vi "JTAG Test App.vi"(1 "Stop Button":bool, 8 "Error In":errorcluster, 11 "Device Name":string="Basys2") -> (0 "Error Out":errorcluster, 3 "ID Codes":u32[](array[numeric]) format="%.0x")   [LabVIEW 2011]
uses:
  Private/DMGR/DMGR.lvlib
  Private/DJTG/DJTG.lvlib
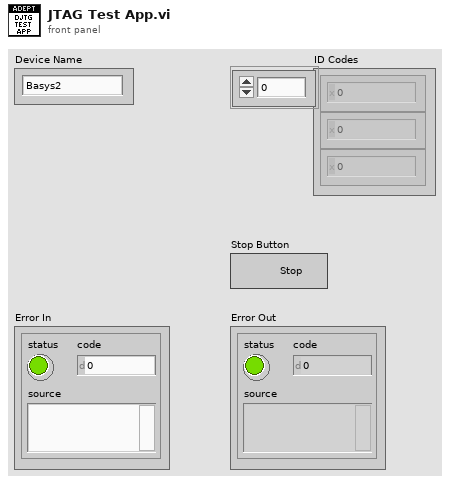
[diagram p1: front panel]
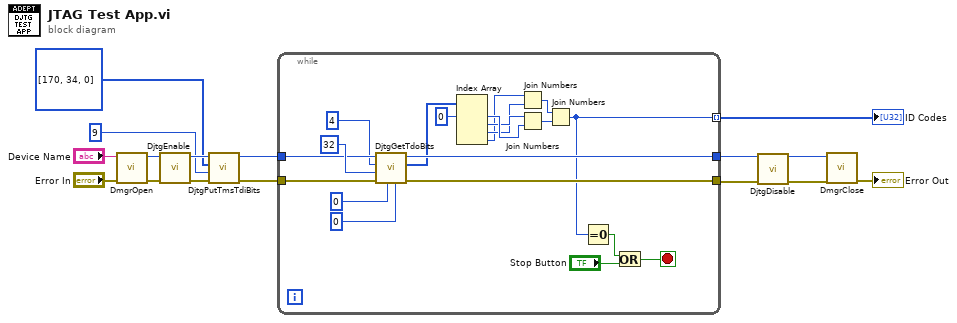
[diagram p0: block diagram]
diagram:
  n1 = call "DmgrOpen.vi"("Error In"="Error In", "Device Name"="Device Name") -> ("Error Out"=w14:errorcluster, "Device Handle"=w13:u32)  [unwired: 8 in]
  n2 = call "DjtgEnable.vi"("Error In"=w14, "Device Number"=w13) -> ("Error Out"=w12:errorcluster, "Device Number"=w11:u32)  [unwired: 8 in]
  n3 = call "DjtgPutTmsTdiBits.vi"("Error In"=w12, "Num Bit Pairs"=u32 9 ("cbitpairs"), "Data To Send"=u8[] [170, 34, 0] ("rgbSnd"), "Device Number"=w11) -> ("Error Out"=w8:errorcluster, "Device Number"=w7:u32)  [unwired: 5 in, 1 out]
  n4 = while {
    tunnel: w8 -> [w36]
    tunnel: w7 -> [w32]
    tunnel: [w31] -> w4
    tunnel: [w30] -> w3
    tunnel: [w20] -> w5 mode=indexing
    stop <- w18 stop-if-true
    n5 = call "DjtgGetTdoBits.vi"("TMS State"=u8 0 ("fTms"), "TDI State"=u8 0 ("fTdi"), "Error In"=w36, "Num Pit Pairs"=u32 32 ("cbitpairs"), "Data Buffer Size (bytes)"=4 ("rgbRec Buffer Size"), "Device Number"=w32) -> ("Error Out"=w30:errorcluster, "Data"=w29:u8[], "Device Number"=w31:u32)  [unwired: 3 in]
    n6 = Index Array(array=w29, index #1=0 ("index")) -> (element #1=w26:u8, element #2=w23:u8, element #3=w22:u8, element #4=w21:u8)  [unwired: 3 in]
    n7 = Join Numbers(hi=w21, lo=w22) -> ((hi.lo)=w24:u16)
    n8 = Join Numbers(hi=w23, lo=w26) -> ((hi.lo)=w25:u16)
    n9 = Join Numbers(hi=w24, lo=w25) -> ((hi.lo)=w20:u32)
    n10 = Equal To 0?(x=w20) -> (x = 0?=w19:bool)
    n11 = Or(x=w19, y="Stop Button") -> (x .or. y?=w18:bool)
  }
  "ID Codes" <- w5
  n12 = call "DjtgDisable.vi"("Error In"=w3, "Device Number"=w4) -> ("Error Out"=w2:errorcluster, "Device Number"=w1:u32)  [unwired: 8 in]
  n13 = call "DmgrClose.vi"("Error In"=w2, "hif"=w1) -> ("Error Out"=→"Error Out":errorcluster)  [unwired: 9 in]
